vi "Publish Case Result.vi"(10 "Test Case Result":refnum<class "Test Case Result.lvclass">, 11 "Slave Test Runner In":refnum<class "Slave Test Runner.lvclass">) -> (3 "Slave Test Runner Out":refnum<class "Slave Test Runner.lvclass">)   [LabVIEW 2020, in "Slave Test Runner.lvclass"]
uses:
  Slave Test Runner.lvclass
  Result Classes/Test Case Result/Test Case Result.lvclass
  Slave Test Runner.lvclass/Slave Test Runner.ctl
  Result Collector/Result Collector.lvclass/Result Collector.ctl
  Result Collector/Result Collector.lvclass
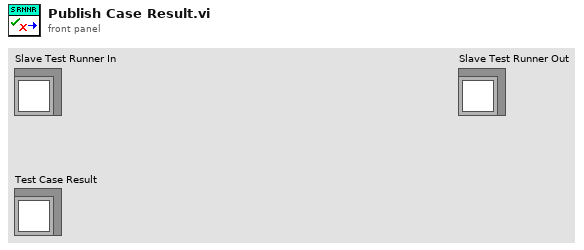
[diagram p1: front panel]
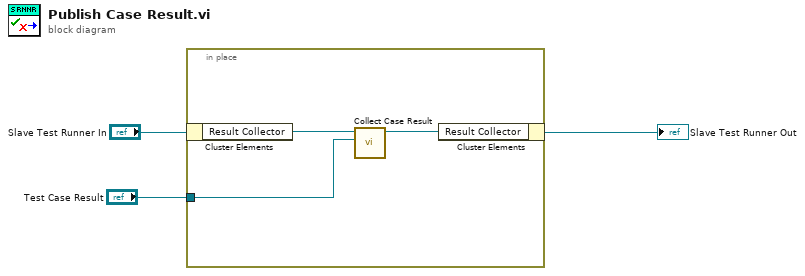
[diagram p0: block diagram]
diagram:
  n1 = in-place {
    in-place-border: "Test Case Result" -> [w4]
    n2 = in-place-cluster #1("Slave Test Runner In") -> ("Result Collector"=w6:refnum<class "Result Collector.lvclass">)
    n3 = call "Collect Case Result.vi"("Test Case Result"=w4, "Report Generator In"=w6) -> ("Report Generator Out"=w5:refnum<class "Result Collector.lvclass">)  [unwired: 9 in]
    n4 = in-place-cluster #1("Result Collector"=w5) -> (→"Slave Test Runner Out":refnum<class "Slave Test Runner.lvclass">)
  }
